vi "UpdateNumericWithScale.vi"(0 "NumericWithScale in":refnum<vi>, 5 "connect":bool, 7 "AI_Data":T1, 11 "error in (no error)":errorcluster) -> (15 "error out":errorcluster)   [LabVIEW 2019]
uses:
  TypeDef/AI_Data.ctl
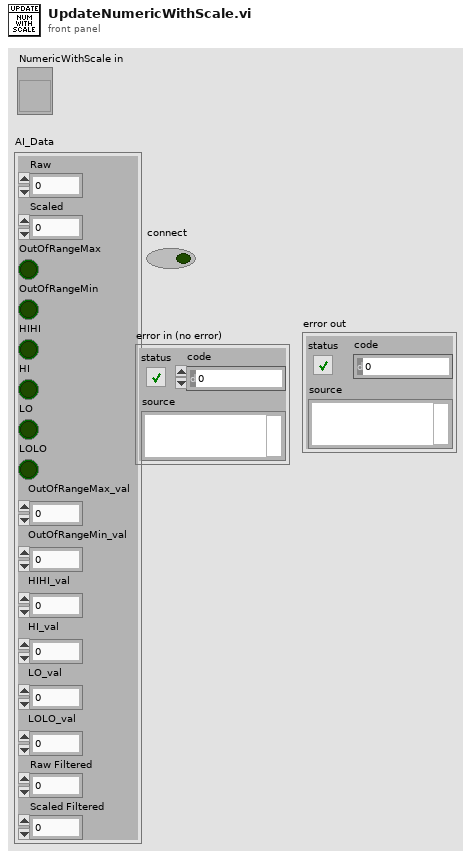
[diagram p1: front panel]
types:
  T1 = typedef "AI_Data.ctl" = cluster{"Raw":dbl, "Scaled":dbl, "OutOfRangeMax":bool, "OutOfRangeMin":bool, "HIHI":bool, "HI":bool, "LO":bool, "LOLO":bool, "OutOfRangeMax_val":dbl, "OutOfRangeMin_val":dbl, "HIHI_val":dbl, "HI_val":dbl, "LO_val":dbl, "LOLO_val":dbl, "Raw Filtered":dbl, "Scaled Filtered":dbl}
  T2 = enum8{"Enabled", "Disabled", "Disabled and Grayed Out"}
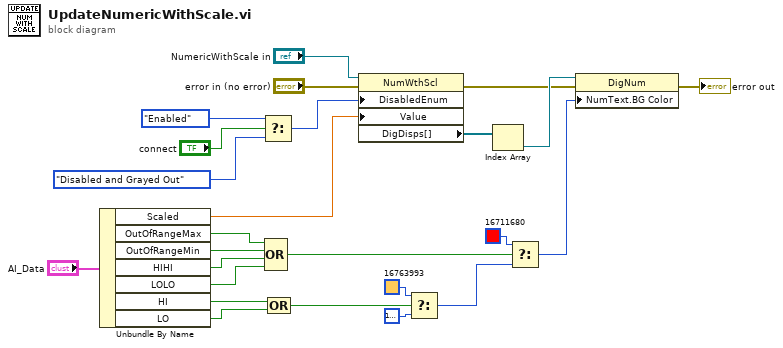
[diagram p0: block diagram]
diagram:
  n1 = Unbundle By Name("AI_Data") -> ("Scaled"=w16:dbl, "OutOfRangeMax"=w15:bool, "OutOfRangeMin"=w14:bool, "HIHI"=w13:bool, "LOLO"=w12:bool, "HI"=w11:bool, "LO"=w10:bool)
  n2 = Select(t=T2."Enabled" ("Disabled"), s="connect", f=T2."Disabled and Grayed Out") -> (s? t:f=w20:T2)
  n3 = Compound Arithmetic op=OR(w15, w14, w13, w12) -> (w4:bool)
  n4 = Compound Arithmetic op=OR(w11, w10) -> (w8:bool)
  n5 = property class="NumWthScl"(reference="NumericWithScale in", error in="error in (no error)", "DisabledEnum"=w20, "Value"=w16) -> (error out=w2:errorcluster, "DigDisps[]"=w19:refnum<vi>[])  [unwired: 1 out]
  n6 = Select(t=u32 16763993 ("Numeric Text.Colors:BG Color"), s=w8, f=u32 16777216 ("Numeric Text.Colors:BG Color")) -> (s? t:f=w6:u32)
  n7 = Index Array(array=w19) -> (element=w18:refnum<vi>)  [unwired: 1 in]
  n8 = Select(t=u32 16711680 ("Numeric Text.Colors:BG Color"), s=w4, f=w6) -> (s? t:f=w3:u32)
  n9 = property class="DigNum"(reference=w18, error in=w2, "NumText.BG Color"=w3) -> (error out=→"error out":errorcluster)  [unwired: 1 out]
